vi "Connection Open.vi"(0 "VISA resource name Out 3":T1={"Conection Data"="COM4"}, 3 "error in (no error)":errorcluster) -> (7 "VISA resource name Out 2":T1={"Conection Data"="COM4"}, 10 "error out":errorcluster)   [LabVIEW 2014, in "AD4212C Lib.lvlib"]
doc: "Abre el puerto COM de la pc colocando el seteado por el usuario y la configuración por defecto que necesita el dispositivo para iniciarse."
uses:
  AD4212C Lib.lvlib
  Typedef/Connection Data.ctl
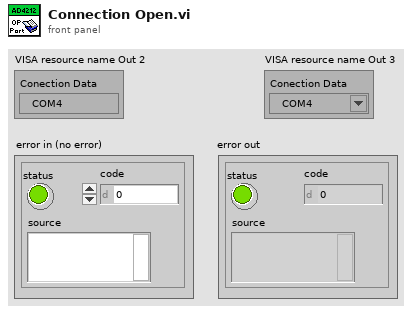
[diagram p1: front panel]
types:
  T1 = typedef "AD4212C Lib.lvlib/Connection Data.ctl" = cluster{"Conection Data":refnum<visa-resource-name>}
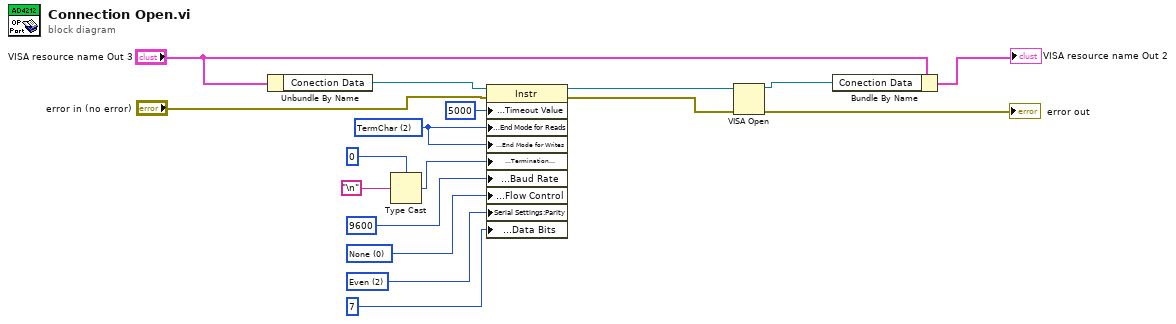
[diagram p0: block diagram]
diagram:
  w6 = u16 2 items=["None", "Odd", "Even", "Mark", "Space"] ("Serial Settings:Parity")
  w7 = u16 0 items=["None", "XON/XOFF", "RTS/CTS", "XON/XOFF & RTS/CTS", "DTR/DSR", "XON/XOFF & DTR/DSR"] ("Serial Settings:Flow Control")
  w9 = u16 2 items=["None", "LastBit", "TermChar"] ("Serial Settings:Serial End Mode for Reads")
  n1 = Unbundle By Name("VISA resource name Out 3") -> ("Conection Data"=w4:refnum<visa-resource-name>)
  n2 = Type Cast(type=u8 0, x="\n") -> (*(type *) &x=w11:u8)
  n3 = property class="Instr"(reference=w4, error in="error in (no error)", "General Settings:Timeout Value"=u32 5000, "Serial Settings:End Mode for Reads"=w9, "Serial Settings:End Mode for Writes"=w9, "Message Based Settings:Termination Character"=w11, "Serial Settings:Baud Rate"=u32 9600, "Serial Settings:Flow Control"=w7, "Serial Settings:Parity"=w6, "Serial Settings:Data Bits"=u16 7) -> (reference out=w14:refnum<visa-resource-name>, error out=w15:errorcluster)
  n4 = VISA Open(error in (no error)=w15, VISA resource name=w14) -> (VISA resource name=w3:refnum<visa-resource-name>, error out=→"error out":errorcluster)  [unwired: 3 in]
  n5 = Bundle By Name(cluster="VISA resource name Out 3", "Conection Data"=w3) -> (→"VISA resource name Out 2":T1)
